vi "Write COMM Status.vi"(8 "error in (no error)":errorcluster, 10 "COMM status":bool, 11 "Hardware in":refnum<class "Hardware.lvclass">) -> (0 "error out":errorcluster, 3 "Hardware out":refnum<class "Hardware.lvclass">)   [LabVIEW 2016, in "Hardware.lvlib" / "Hardware.lvclass"]
uses:
  <userlib>/Common Components/Hardware/Abstract Hardware/Hardware.lvclass
  <userlib>/Common Components/Hardware/Abstract Hardware/Hardware.lvclass/Hardware.ctl
  <userlib>/Common Components/Hardware/DevInfo/DevInfo.lvclass/DevInfo.ctl
  <userlib>/Common Components/Hardware/DevInfo/Write Status.vi
  <userlib>/Common Components/Hardware/DevInfo/DevInfo.lvclass
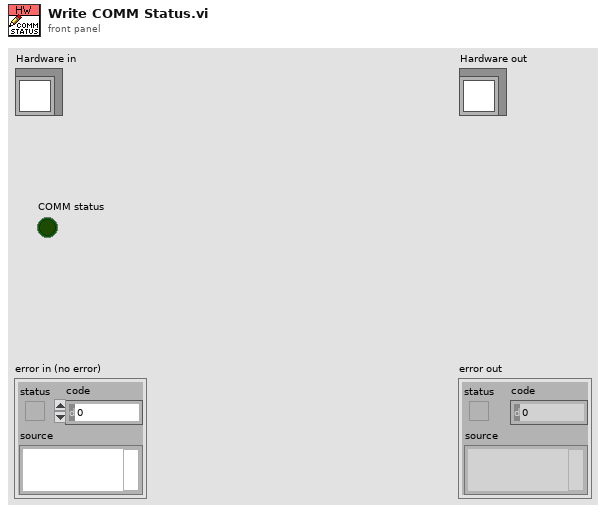
[diagram p1: front panel]
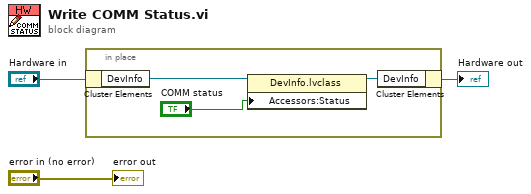
[diagram p0: block diagram]
diagram:
  n1 = in-place {
    n2 = in-place-cluster #1("Hardware in") -> ("DevInfo"=w6:refnum<class "DevInfo.lvclass">)
    n3 = property class="DevInfo.lvclass"(reference=w6, "Accessors:Status"="COMM status") -> (reference out=w5:refnum<class "DevInfo.lvclass">)  [unwired: 1 in, 1 out]
    n4 = in-place-cluster #1("DevInfo"=w5) -> (→"Hardware out":refnum<class "Hardware.lvclass">)
  }
  "error out" <- "error in (no error)"
